vi "Read Register.vi"(8 "error in (no error)":errorcluster, 10 "Register":u8 format="%.0x", 11 "VISA resource name":refnum<visa-resource-name>) -> (0 "error out":errorcluster, 2 "Value":u8 format="%x", 3 "VISA resource name out":refnum<visa-resource-name>)   [LabVIEW 2013, in "HadCon.lvlib"]
doc: "Read register value."
uses:
  <instrlib>/HadCon/HadCon.lvlib
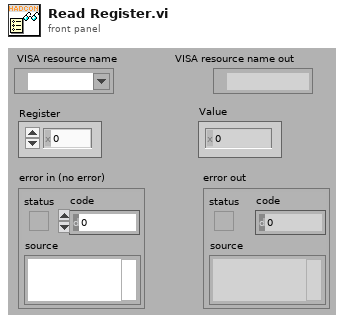
[diagram p1: front panel]
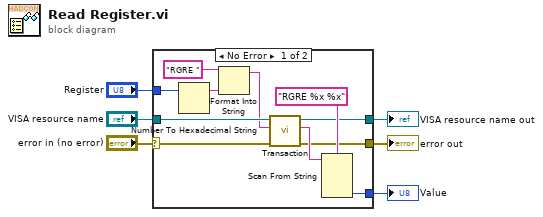
[diagram p0: block diagram]
diagram:
  n1 = case shown="No Error" "error in (no error)" {
    selector: "error in (no error)" -> [w13 w18]
    tunnel: [w8 w19] -> w6
    tunnel: "VISA resource name" -> [w17 w19]
    tunnel: [w7 w18] -> w4
    tunnel: "Register" -> [w15 _]
    tunnel: [w10 _] -> w1
    frame No Error {
      n2 = Number To Hexadecimal String(2:w15) -> (0:w9:string)  [unwired: 1 in]
      n3 = Format Into String(initial string="RGRE ", w9) -> (resulting string=w14:string)  [unwired: 2 in, 1 out]
      n4 = call <instrlib>:"Transaction.vi"("Error In"=w13, "Command"=w14, "VISA resource name"=w17) -> ("Error Out"=w7:errorcluster, "Response"=w12:string, "VISA resource name out"=w8:refnum<visa-resource-name>)  [unwired: 6 in]
      n5 = Scan From String(format string="RGRE %x %x", input string=w12) -> (output 2=w10:u32)  [unwired: 5 in, 3 out]
    }
    frame Error {
    }
  }
  "VISA resource name out" <- w6
  "error out" <- w4
  "Value" <- w1
